vi "1.6.vi"() -> ()   [LabVIEW 2017]
panel:
  out "String 2":string
  in  "Integer":dbl
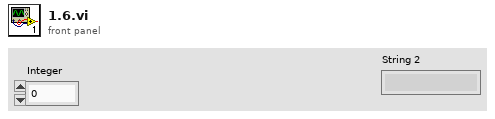
[diagram p1: front panel]
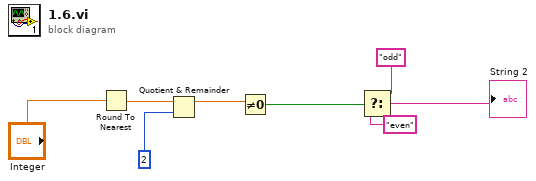
[diagram p0: block diagram]
diagram:
  n1 = Round To Nearest(number="Integer") -> (nearest integer value=w6:dbl)
  n2 = Quotient & Remainder(x=w6, y=2) -> (x-y*floor(x/y)=w7:dbl)  [unwired: 1 out]
  n3 = Not Equal To 0?(x=w7) -> (x != 0?=w4:bool)
  n4 = Select(t="odd", s=w4, f="even") -> (s? t:f=→"String 2":string)
